vi "SMU.GetCurrent.vi"(8 "error in (no error)":errorcluster, 11 "SMU.Keithley2600 in":refnum<class "SMU.Keithley2600.lvclass">) -> (0 "error out":errorcluster, 2 "Current, A":dbl format="%#_13g", 3 "SMU.Keithley2600 out":refnum<class "SMU.Keithley2600.lvclass">)   [LabVIEW 2017, in "SMU.Keithley2600.lvclass"]
uses:
  SMU.Keithley2600.lvclass
  <instrlib>/Keithley 2600 Series/Public/Data/Read Measurement (Current).vi
  <instrlib>/Keithley 2600 Series/Keithley 2600 Series.lvlib
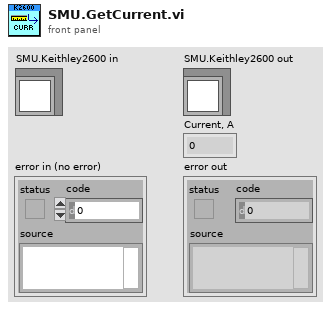
[diagram p1: front panel]
types:
  T1 = typedef "SMU.Keithley2600.lvclass/Resource--Cluster.ctl" = cluster{"VISA resource":refnum<visa-resource-name>, "Channel":i32}
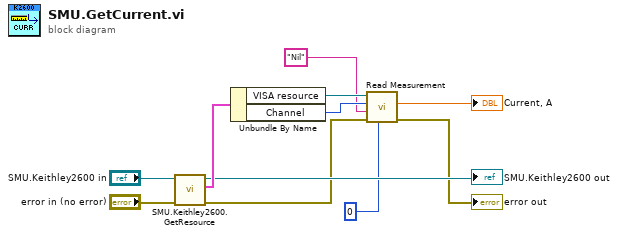
[diagram p0: block diagram]
diagram:
  n1 = call "SMU.Keithley2600.GetResource.vi"("error in (no error)"="error in (no error)", "SMU.Keithley2600 in"="SMU.Keithley2600 in") -> ("error out"=w5:errorcluster, "Resource"=w9:T1, "SMU.Keithley2600 out"=→"SMU.Keithley2600 out":refnum<class "SMU.Keithley2600.lvclass">)  [unwired: 7 in]
  n2 = Unbundle By Name(w9) -> ("VISA resource"=w7:refnum<visa-resource-name>, "Channel"=w6:i32)
  n3 = call-poly <instrlib>:"Read Measurement.vi"("Wait Time (10 S)"=0, "error in (no error)"=w5, "Current Buffer (smua.nvbuffer1)"="Nil", "Source Measure Unit Channel (0: Channel A)"=w6, "VISA resource name"=w7) -> ("error out"=→"error out":errorcluster, "Last Current (A)"=→"Current, A":dbl)  [unwired: 3 in, 2 out]
